vi "DecodeNTType.vi"(11 "string":string) -> (0 "string":string, 1 "boolean":bool, 2 "number":dbl, 3 "type":string)   [LabVIEW 2012]
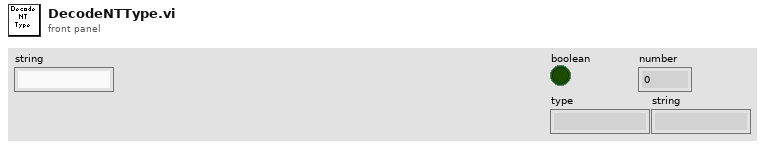
[diagram p1: front panel]
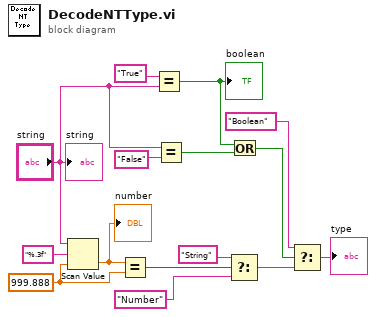
[diagram p0: block diagram]
diagram:
  w13 = 999.888 ("default (0 dbl)")
  n1 = Scan Value(string="string", format string="%.3f", default (0 dbl)=w13) -> (value=w14:dbl)  [unwired: 1 out]
  "number" <- w14
  n2 = Equal?(x=w14, y=w13) -> (x = y?=w10:bool)
  n3 = Equal?(x="True" ("string"), y="string") -> (x = y?=w6:bool)
  "boolean" <- w6
  n4 = Equal?(x="string", y="False" ("true string")) -> (x = y?=w7:bool)
  n5 = Select(t="String" ("true string"), s=w10, f="Number") -> (s? t:f=w3:string)
  n6 = Or(x=w6, y=w7) -> (x .or. y?=w5:bool)
  n7 = Select(t="Boolean" ("string"), s=w5, f=w3) -> (s? t:f=→"type":string)
  "string" <- "string"
